vi "CRYFind Same Name.vi"(10 "Name":string, 11 "sNames":string[](array[string])) -> (0 "bResult":bool, 2 "NameOut":string, 3 "Index":i32)   [LabVIEW 2013]
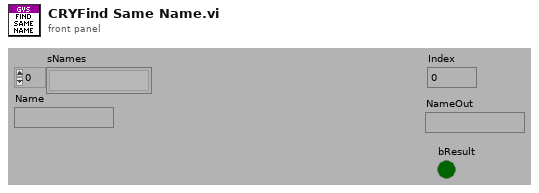
[diagram p1: front panel]
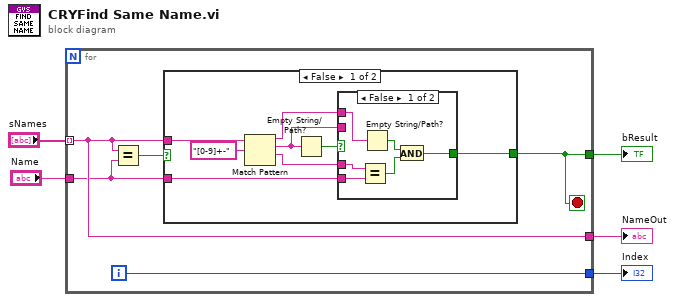
[diagram p0: block diagram]
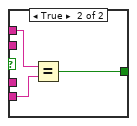
[diagram p2: hidden frame]
diagram:
  n1 = for {
    tunnel: "sNames" -> [w8] mode=indexing
    tunnel: "Name" -> [w7]
    tunnel: [w10] -> w2
    tunnel: [w9] -> w3
    tunnel: [w8] -> w1
    i -> [w10]
    stop <- w9 stop-if-true
    n2 = Equal?(x=w8, y=w7) -> (x = y?=w6:bool)
    n3 = case shown="False" w6 {
      selector: w6 -> [_ w28]
      tunnel: w7 -> [w14 _]
      tunnel: [w13 w28] -> w9
      tunnel: w8 -> [w11 _]
      frame False {
        n4 = Match Pattern(string=w11, regular expression="[0-9]+-") -> (before substring=w15:string, match substring=w16:string, after substring=w12:string)  [unwired: 1 in, 1 out]
        n5 = Empty String/Path?(string/path=w16) -> (empty?=w17:bool)
        n6 = case shown="False" w17 {
          tunnel: w16 -> [_ _]
          tunnel: w14 -> [w24 w27]
          tunnel: w12 -> [w23 _]
          tunnel: w15 -> [w22 w25]
          tunnel: [w19 w26] -> w13
          frame False {
            n7 = Equal?(x=w23, y=w24) -> (x = y?=w20:bool)
            n8 = Empty String/Path?(string/path=w22) -> (empty?=w21:bool)
            n9 = And(x=w21, y=w20) -> (x .and. y?=w19:bool)
          }
          frame True {
            n10 = Equal?(x=w25, y=w27) -> (x = y?=w26:bool)
          }
        }
      }
      frame True {
      }
    }
  }
  "bResult" <- w3
  "Index" <- w2
  "NameOut" <- w1
